vi "simulador_temperatura.vi"(1 "L max":dbl, 2 "Lmini":dbl) -> (0 "Numeric":dbl)   [LabVIEW 2020]
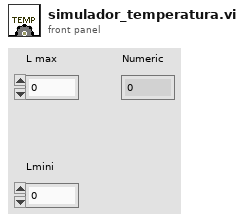
[diagram p1: front panel]
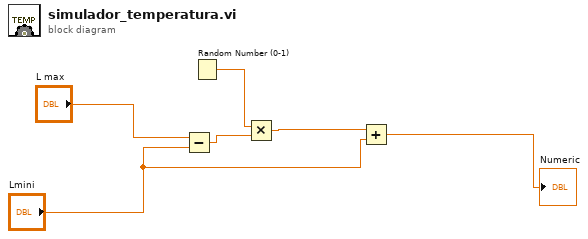
[diagram p0: block diagram]
diagram:
  n1 = Subtract(x="L max", y="Lmini") -> (x-y=w2:dbl)
  n2 = Random Number (0-1)() -> (number: 0 to 1=w3:dbl)
  n3 = Multiply(x=w3, y=w2) -> (x*y=w4:dbl)
  n4 = Add(x=w4, y="Lmini") -> (x+y=→"Numeric":dbl)
